vi "Get FKV Shift Speed.vi"(10 "speed":i32, 11 "index":i32) -> (2 "speed out":i32, 3 "function return":u32)   [LabVIEW 2018, in "Copy of Andor SDK.lvlib"]
doc: "EXPNETTYPE unsigned int WINAPI GetFKVShiftSpeed(int index, int * speed);"
uses:
  Copy of Andor SDK.lvlib
  <userlib>/Andor SDK/ATMCD32D.dll
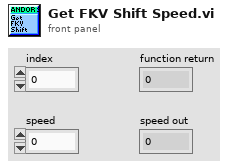
[diagram p1: front panel]
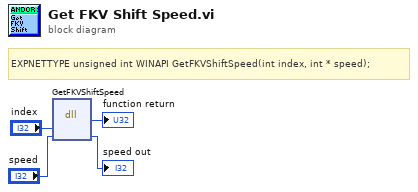
[diagram p0: block diagram]
diagram:
  # "EXPNETTYPE unsigned int WINAPI GetFKVShiftSpeed(int index, int * speed);"
  n1 = dll-call lib="C:/Program Files (x86)/National Instruments/LabVIEW 2018/user.lib/Andor SDK/ATMCD32D.*" fn="GetFKVShiftSpeed"("index"="index", "speed"="speed") -> (→"function return":u32, "speed"=→"speed out":i32)  [unwired: 4 in, 2 out]
